vi "Idle_ProbeWeatherStation.vi"(0 "IP Address":string="192.168.0.110", 1 "Working Directory":path=path "C:/Users/h2odial/WVD-MCSupdate/WVDNewArchitectureUpdate/WVD_Architecture_Update/NetCDFPython/SocketComms", 2 "PathToPython":string="C:\\Users\\h2odial\\Anaconda3\\python.exe", 3 "PathToScript":string="CallWeatherStation.py", 5 "Port":i32=4760, 7 "Timeout [ms]":i32=1000, 11 "ErrorIn":errorcluster) -> (4 "PythonResponse":string="WS_Luft_WSData_-2001_-2001_-2001_-2001\r\n", 6 "StandardError":string, 15 "ErrorOut":errorcluster)   [LabVIEW 2024]
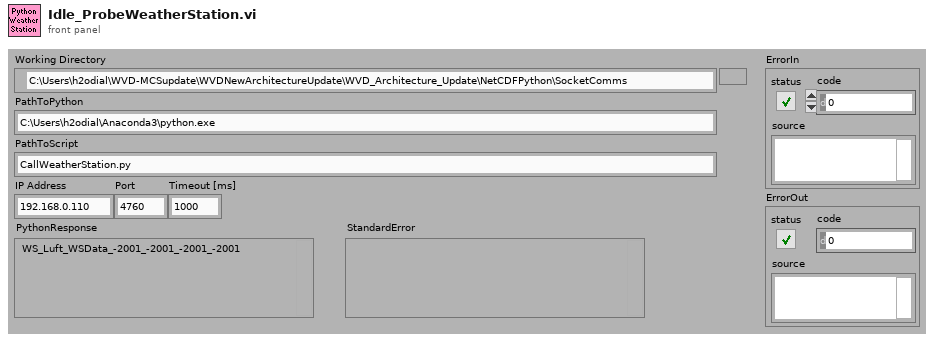
[diagram p1: front panel]
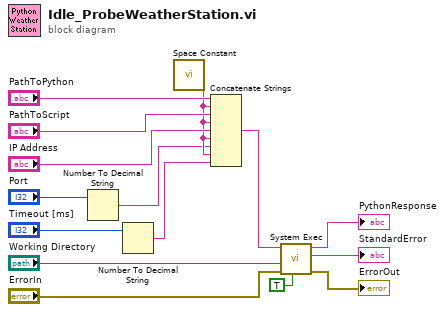
[diagram p0: block diagram]
diagram:
  n1 = Number To Decimal String(number="Port") -> (decimal integer string=w2:string)  [unwired: 1 in]
  n2 = Number To Decimal String(number="Timeout [ms]") -> (decimal integer string=w1:string)  [unwired: 1 in]
  n3 = call <vilib>:"Space Constant.vi"() -> ("String"=w6:string)
  n4 = Concatenate Strings("PathToPython", w6, "PathToScript", w6, "IP Address", w6, w2, w6, w1) -> (w14:string)
  n5 = call <vilib>:"System Exec.vi"("run minimized? (F)"=TRUE, "error in (no error)"="ErrorIn", "working directory"="Working Directory", "command line"=w14) -> ("error out"=→"ErrorOut":errorcluster, "standard error"=→"StandardError":string, "standard output"=→"PythonResponse":string)  [unwired: 2 in, 3 out]
